vi "Handle Error.vi"(8 "error in (no error)":errorcluster, 11 "Measurement UI in":refnum<class "Measurement UI.lvclass">) -> (0 "error out":errorcluster, 2 "stop actor?":bool=TRUE, 3 "Measurement UI out":refnum<class "Measurement UI.lvclass">)   [LabVIEW 2015, in "Measurement UI.lvlib" / "Measurement UI.lvclass"]
doc: "(<B>Filename</B>: Actor Framework.lvlib:Actor.lvclass:Handle Error.vi)\n\nDefines how the actor handles an error that occurred while processing a message.\n\nBy default, this method does nothing except stop the actor. This method also treats error code 43 (coming from <B>error in</B>) as a sign that the actor shut down normally. In this situation, the Handle Error method does not return the error on <B>error out</B>, meaning the actor's caller will not receive it. All other error codes will be returned on <B>error out</B>.\n\nA descendant class may override this method to change this behavior."
uses:
  Measurement UI.lvclass
  <vilib>/ActorFramework/Actor/Actor.lvclass/Actor.ctl
  <vilib>/ActorFramework/Message Enqueuer/Message Enqueuer.lvclass/Message Enqueuer.ctl
  <vilib>/ActorFramework/Message Enqueuer/Init from Existing Queue.vi
  <vilib>/ActorFramework/Message Enqueuer/Message Enqueuer.lvclass
  User Interface/UI.lvclass
  User Interface/Messages/Update Status Display/Update Status Display.lvclass
  <vilib>/ActorFramework/Actor/Actor.lvclass
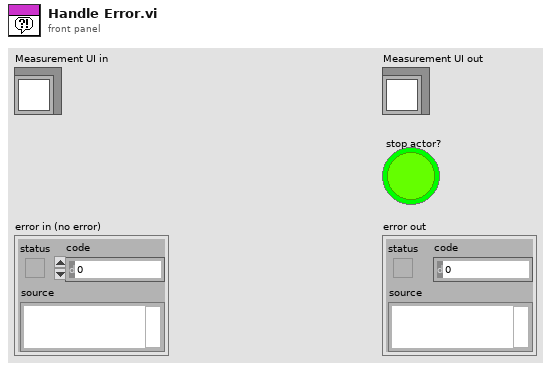
[diagram p1: front panel]
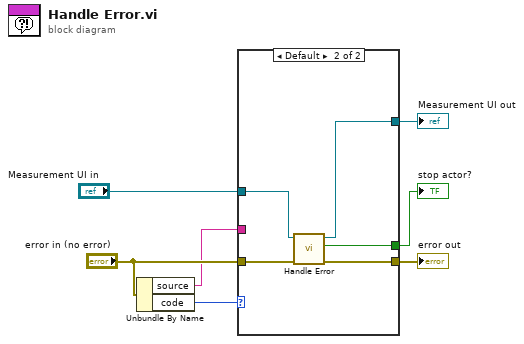
[diagram p0: block diagram]
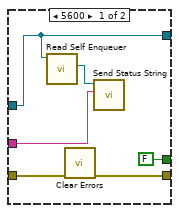
[diagram p2: hidden frame]
diagram:
  n1 = Unbundle By Name("error in (no error)") -> ("source"=w1:string, "code"=w2:i32)
  n2 = case shown="Default" w2 {
    tunnel: [w11 w18] -> w7
    tunnel: [FALSE ("stop actor?") w17] -> w6
    tunnel: [w10 w16] -> w5
    tunnel: "error in (no error)" -> [w12 w15]
    tunnel: "Measurement UI in" -> [w10 w14]
    tunnel: w1 -> [w8 _]
    frame 5600 {
      n3 = call <vilib>:"Read Self Enqueuer.vi"("Actor"=w10) -> ("Self Enqueuer"=w9:refnum<class "Message Enqueuer.lvclass">)  [unwired: 10 in]
      n4 = call <vilib>:"Clear Errors.vi"("error in (no error)"=w12) -> ("error out"=w11:errorcluster)  [unwired: 5 in, 1 out]
      n5 = call "Send Status String.vi"("String"=w8, "Message Enqueuer in"=w9) -> ()  [unwired: 8 in, 2 out]
    }
    frame Default {
      n6 = call-parent "Handle Error.vi"("error in (no error)"=w15, "Actor in"=w14) -> ("error out"=w18:errorcluster, "stop actor?"=w17:bool, "Actor out"=w16:refnum<class "Measurement UI.lvclass">)  [unwired: 7 in]
    }
  }
  "Measurement UI out" <- w5
  "error out" <- w7
  "stop actor?" <- w6
